vi "Strip To.vi"(6 "End":string, 8 "error in (no error)":errorcluster, 10 "String":string, 11 "ProtoParser in":refnum<class "ProtoParser.lvclass">) -> (0 "error out":errorcluster, 1 "Portion":string, 2 "Remaining":string, 3 "ProtoParser out":refnum<class "ProtoParser.lvclass">)   [LabVIEW 2020, in "LV-Protoc.lvlib" / "ProtoParser.lvclass"]
uses:
  ProtoParser.lvclass
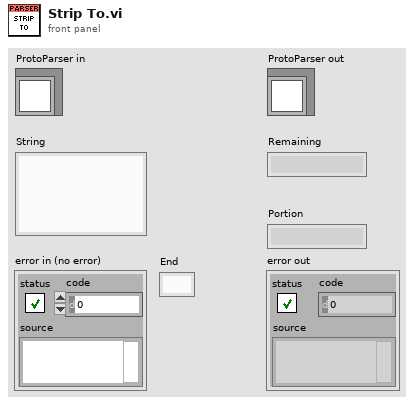
[diagram p1: front panel]
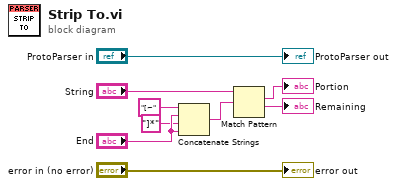
[diagram p0: block diagram]
diagram:
  n1 = Concatenate Strings("[~" ("string"), "End", "]*" ("string"), "End") -> (w1:string)
  n2 = Match Pattern(string="String", regular expression=w1) -> (match substring=→"Portion":string, after substring=→"Remaining":string)  [unwired: 1 in, 2 out]
  "error out" <- "error in (no error)"
  "ProtoParser out" <- "ProtoParser in"
